vi "Read DIO signals.vi"(8 "error in (no error)":errorcluster) -> (0 "error out":errorcluster, 3 "Relays":T1)   [LabVIEW 2025]
uses:
  Controls/DUT_Relays.ctl
  Controls/CHMB_Relays.ctl
  Controls/Relays.ctl
  <vilib>/Utility/config.llb/Read Key (U32).vi
  <vilib>/Utility/config.llb/NI_LVConfig.lvlib
panel:
  out "CHMB2":T2
  out "CHMB1":T2
  out "DUT4":T3
  out "DUT3":T3
  out "DUT2":T3
  out "DUT1":T3
  out "error IO":errorcluster
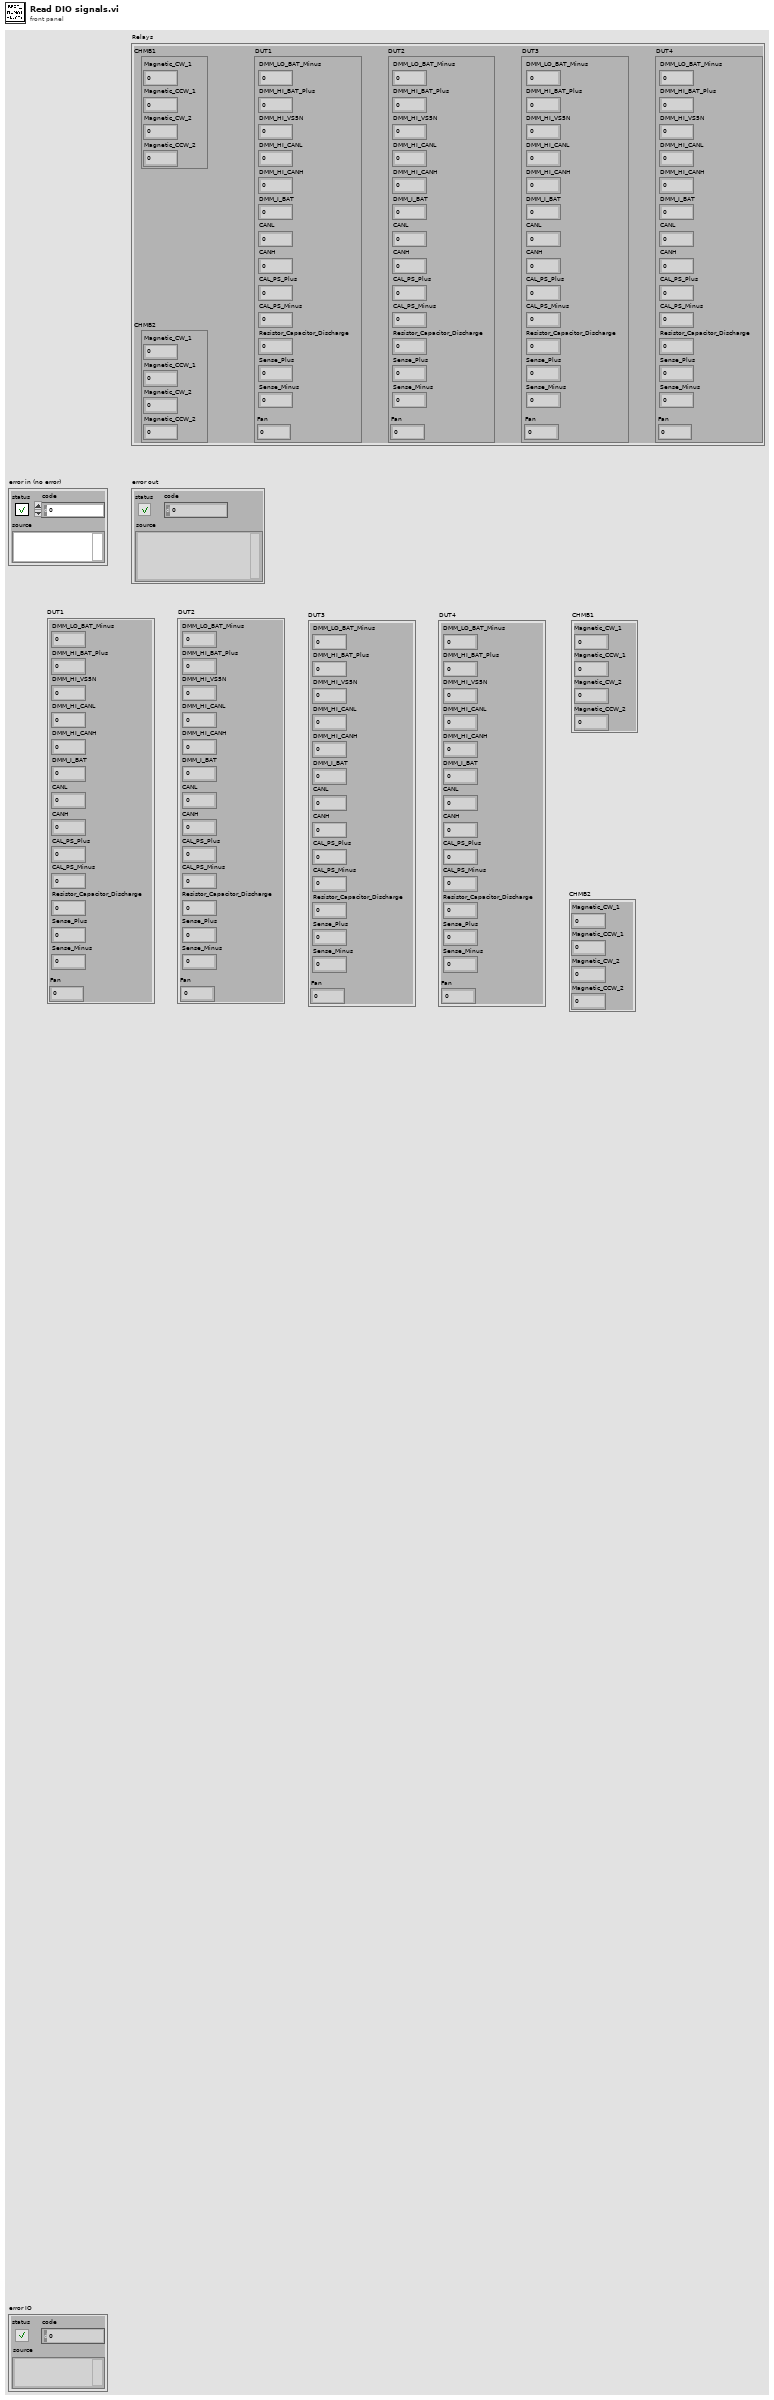
[diagram p1: front panel]
types:
  T1 = typedef "Relays.ctl" = cluster{"CHMB1":T2, "CHMB2":T2, "DUT1":T3, "DUT2":T3, "DUT3":T3, "DUT4":T3}
  T2 = typedef "CHMB_Relays.ctl" = cluster{"Magnetic_CW_1":i32, "Magnetic_CCW_1":i32, "Magnetic_CW_2":i32, "Magnetic_CCW_2":i32}
  T3 = typedef "DUT_Relays.ctl" = cluster{"DMM_LO_BAT_Minus":i32, "DMM_HI_BAT_Plus":i32, "DMM_HI_VS5N":i32, "DMM_HI_CANL":i32, "DMM_HI_CANH":i32, "DMM_I_BAT":i32, "CANL":i32, "CANH":i32, "CAL_PS_Plus":i32, "CAL_PS_Minus":i32, "Resistor_Capacitor_Discharge":i32, "Sense_Plus":i32, "Sense_Minus":i32, "Fan":i32}
  T4 = typedef "NI_LVConfig.lvlib/Config Data RefNum.ctl" = refnum<k1>
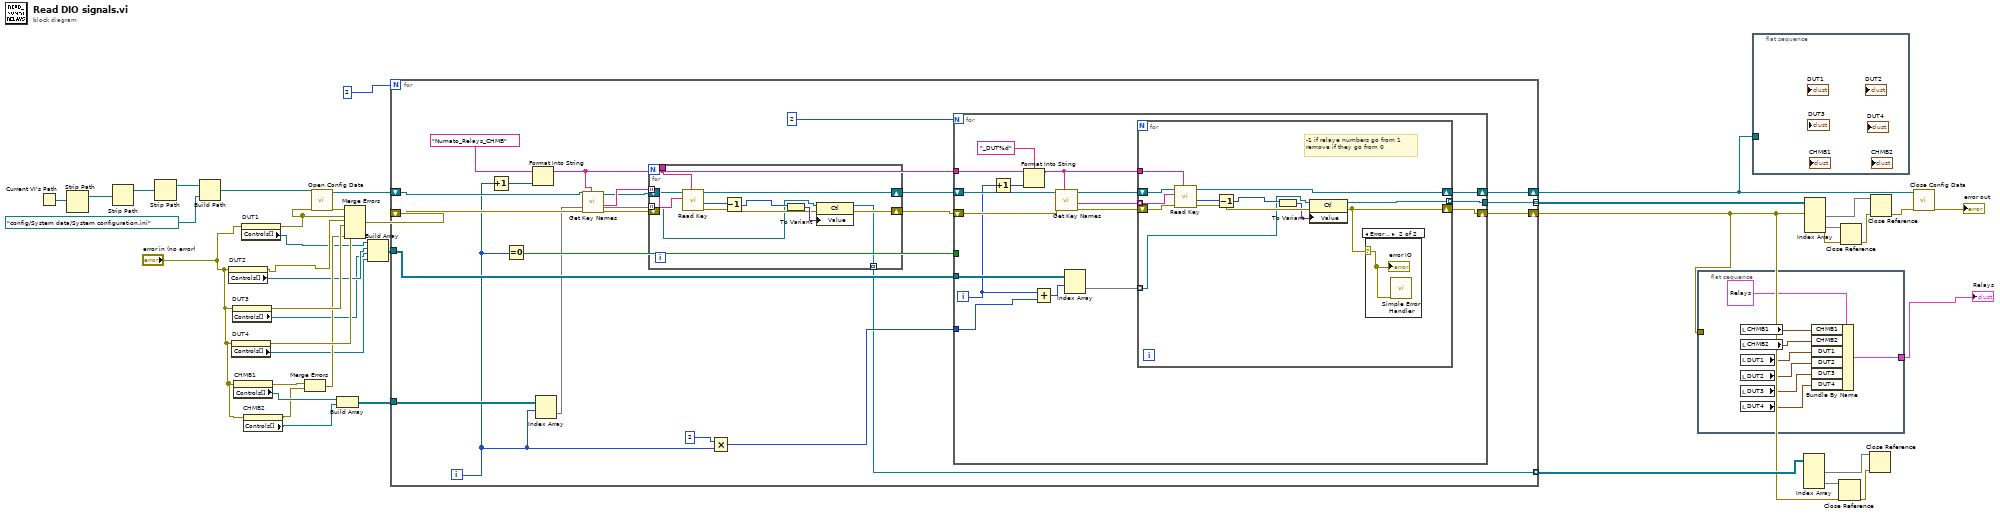
[diagram p0: block diagram]
diagram:
  n1 = Current VI's Path() -> (path=w26:path)
  n2 = Strip Path(path=w26) -> (stripped path=w25:path)  [unwired: 1 out]
  n3 = Strip Path(path=w25) -> (stripped path=w29:path)  [unwired: 1 out]
  n4 = Strip Path(path=w29) -> (stripped path=w28:path)  [unwired: 1 out]
  n5 = Build Path(base path=w28, name or relative path=path "config/System data/System configuration.ini") -> (appended path=w24:path)
  n6 = property on="DUT2" class="Clust (strict)"(error in="error in (no error)") -> (error out=w22:errorcluster, "Controls[]"=w16:refnum<vi>[])  [unwired: 1 in, 1 out]
  n7 = property on="DUT4" class="Clust (strict)"(error in="error in (no error)") -> (error out=w19:errorcluster, "Controls[]"=w14:refnum<vi>[])  [unwired: 1 in, 1 out]
  n8 = property on="DUT3" class="Clust (strict)"(error in="error in (no error)") -> (error out=w20:errorcluster, "Controls[]"=w15:refnum<vi>[])  [unwired: 1 in, 1 out]
  n9 = property on="CHMB1" class="Clust (strict)"(error in="error in (no error)") -> (error out=w21:errorcluster, "Controls[]"=w12:refnum<vi>[])  [unwired: 1 in, 1 out]
  n10 = property on="DUT1" class="Clust (strict)"(error in="error in (no error)") -> (error out=w23:errorcluster, "Controls[]"=w17:refnum<vi>[])  [unwired: 1 in, 1 out]
  n11 = property on="CHMB2" class="Clust (strict)"(error in="error in (no error)") -> (error out=w5:errorcluster, "Controls[]"=w4:refnum<vi>[])  [unwired: 1 in, 1 out]
  n12 = Merge Errors(w21, w5) -> (w18:errorcluster)
  n13 = call <vilib>:"Open Config Data.vi"("error in (no error)"=w23, "configuration file path"=w24) -> ("error out"=w34:errorcluster, "refnum"=w39:T4)  [unwired: 7 in, 1 out]
  n14 = Build Array(w12, w4) -> (w11:refnum<vi>[][])
  n15 = Merge Errors(w34, w23, w22, w20, w19, w18) -> (w35:errorcluster)
  n16 = Build Array(w17, w16, w15, w14) -> (w13:refnum<vi>[][])
  n17 = for {
    N: 2 -> [_]
    shift-right: [w60] -> w3
    shift-left: w39 -> [w55]
    shift-right: [w61] -> w2
    shift-left: w35 -> [w54]
    tunnel: [w57] -> w33 mode=indexing
    tunnel: w13 -> [w52]
    tunnel: w11 -> [w50]
    tunnel: [w41] -> w10 mode=indexing
    i -> [w40]
    n18 = Increment(x=w40) -> (x+1=w51:i32)
    n19 = Equal To 0?(x=w40) -> (x = 0?=w58:bool)
    n20 = Format Into String(initial string="Numato_Relays_CHMB" ("section"), w51) -> (resulting string=w46:string)  [unwired: 2 in, 1 out]
    n21 = Index Array(array=w50, index (row)=w40) -> (element=w49:refnum<vi>[])  [unwired: 1 in]
    n22 = call <vilib>:"Get Key Names.vi"("section"=w46, "error in (no error)"=w54, "refnum"=w55) -> ("error out"=w44:errorcluster, "key names"=w53:string[], "refnum out"=w43:T4)  [unwired: 5 in, 1 out]
    n23 = for {
      tunnel: w53 -> [w68] mode=indexing
      tunnel: w49 -> [w66] mode=indexing
      tunnel: w46 -> [w67]
      shift-right: [w65] -> w45
      shift-left: w44 -> [_]
      shift-right: [w63] -> w42
      shift-left: w43 -> [w64]
      tunnel: [w62] -> w41 mode=indexing
      n24 = call-poly <vilib>:"Read Key.vi"("section"=w67, "key"=w68, "refnum"=w64) -> ("error out"=w69:errorcluster, "value"=w70:u32, "refnum out"=w63:T4)  [unwired: 5 in, 1 out]
      n25 = Decrement(x=w70) -> (x-1=w71:u32)
      n26 = To Variant(anything=w71) -> (Variant=w72:variant)
      n27 = property class="Ctl"(reference=w66, error in=w69, "Value"=w72) -> (reference out=w62:refnum<vi>, error out=w65:errorcluster)
    }
    n28 = Multiply(x=2, y=w40) -> (x*y=w47:i32)
    n29 = for {
      N: 2 -> [_]
      tunnel: w58 -> [_]
      tunnel: [w83] -> w57
      shift-right: [w84] -> w60
      shift-left: w42 -> [w89]
      shift-right: [w85] -> w61
      shift-left: w45 -> [w87]
      tunnel: w46 -> [w81]
      tunnel: w52 -> [w78]
      tunnel: w47 -> [w75]
      i -> [w73]
      n30 = Increment(x=w73) -> (x+1=w76:i32)
      n31 = Format Into String(format string="_DUT%d", initial string=w81, w76) -> (resulting string=w80:string)  [unwired: 1 in, 1 out]
      n32 = Add(x=w73, y=w75) -> (x+y=w74:i32)
      n33 = call <vilib>:"Get Key Names.vi"("section"=w80, "error in (no error)"=w87, "refnum"=w89) -> ("error out"=w86:errorcluster, "key names"=w82:string[], "refnum out"=w88:T4)  [unwired: 5 in, 1 out]
      n34 = Index Array(array=w78, index (row)=w74) -> (element=w77:refnum<vi>[])  [unwired: 1 in]
      n35 = for {
        tunnel: w82 -> [w99] mode=indexing
        shift-right: [w100] -> w84
        shift-left: w88 -> [w101]
        tunnel: w80 -> [w98]
        tunnel: [w95] -> w83 mode=indexing
        shift-right: [w94] -> w85
        shift-left: w86 -> [w97]
        tunnel: w77 -> [w91] mode=indexing
        # "-1 if relaye numbers go from 1\nremove if they go from 0"
        n36 = call-poly <vilib>:"Read Key.vi"("section"=w98, "error in (no error)"=w97, "key"=w99, "refnum"=w101) -> ("error out"=w96:errorcluster, "value"=w93:u32, "refnum out"=w100:T4)  [unwired: 4 in, 1 out]
        n37 = Decrement(x=w93) -> (x-1=w92:u32)
        n38 = To Variant(anything=w92) -> (Variant=w90:variant)
        n39 = property class="Ctl"(reference=w91, error in=w96, "Value"=w90) -> (reference out=w95:refnum<vi>, error out=w94:errorcluster)
        n40 = case shown="Error .." w94 {
          selector: w94 -> [_ w102]
          frame No Error {
          }
          frame Error {
            n41 = call <vilib>:"Simple Error Handler.vi"("error in (no error)"=w102) -> ()  [unwired: 4 in, 5 out]
            "error IO" <- w102
          }
        }
      }
    }
  }
  n42 = flat-sequence {
    tunnel: w2 -> [_]
    tunnel: [w104] -> w1
    frame #0 {
      n43 = local read "CHMB1"() -> (w109:T2)
      n44 = local read "CHMB2"() -> (w103:T2)
      n45 = local read "DUT1"() -> (w108:T3)
      n46 = local read "DUT2"() -> (w107:T3)
      n47 = local read "DUT3"() -> (w106:T3)
      n48 = local read "DUT4"() -> (w105:T3)
      n49 = Bundle By Name(cluster=T1 {"CHMB1"={"Magnetic_CW_1"=0, "Magnetic_CCW_1"=0, "Magnetic_CW_2"=0, "Magnetic_CCW_2"=0}, "CHMB2"={"Magnetic_CW_1"=0, "Magnetic_CCW_1"=0, "Magnetic_CW_2"=0, "Magnetic_CCW_2"=0}, "DUT1"={"DMM_LO_BAT_Minus"=0, "DMM_HI_BAT_Plus"=0, "DMM_HI_VS5N"=0, "DMM_HI_CANL"=0, "DMM_HI_CANH"=0, "DMM_I_BAT"=0, "CANL"=0, "CANH"=0, "CAL_PS_Plus"=0, "CAL_PS_Minus"=0, "Resistor_Capacitor_Discharge"=0, "Sense_Plus"=0, "Sense_Minus"=0, "Fan"=0}, "DUT2"={"DMM_LO_BAT_Minus"=0, "DMM_HI_BAT_Plus"=0, "DMM_HI_VS5N"=0, "DMM_HI_CANL"=0, "DMM_HI_CANH"=0, "DMM_I_BAT"=0, "CANL"=0, "CANH"=0, "CAL_PS_Plus"=0, "CAL_PS_Minus"=0, "Resistor_Capacitor_Discharge"=0, "Sense_Plus"=0, "Sense_Minus"=0, "Fan"=0}, "DUT3"={"DMM_LO_BAT_Minus"=0, "DMM_HI_BAT_Plus"=0, "DMM_HI_VS5N"=0, "DMM_HI_CANL"=0, "DMM_HI_CANH"=0, "DMM_I_BAT"=0, "CANL"=0, "CANH"=0, "CAL_PS_Plus"=0, "CAL_PS_Minus"=0, "Resistor_Capacitor_Discharge"=0, "Sense_Plus"=0, "Sense_Minus"=0, "Fan"=0}, "DUT4"={"DMM_LO_BAT_Minus"=0, "DMM_HI_BAT_Plus"=0, "DMM_HI_VS5N"=0, "DMM_HI_CANL"=0, "DMM_HI_CANH"=0, "DMM_I_BAT"=0, "CANL"=0, "CANH"=0, "CAL_PS_Plus"=0, "CAL_PS_Minus"=0, "Resistor_Capacitor_Discharge"=0, "Sense_Plus"=0, "Sense_Minus"=0, "Fan"=0}} ("Relays"), "CHMB1"=w109, "CHMB2"=w103, "DUT1"=w108, "DUT2"=w107, "DUT3"=w106, "DUT4"=w105) -> (w104:T1)
    }
  }
  n50 = flat-sequence {
    tunnel: w3 -> [_]
    frame #0 {
    }
  }
  n51 = Index Array(array=w10) -> (element #1=w7:refnum<vi>[], element #2=w8:refnum<vi>[])  [unwired: 4 in]
  n52 = Index Array(array=w33) -> (element #1=w32:refnum<vi>[], element #2=w31:refnum<vi>[])  [unwired: 4 in]
  n53 = Close Reference(reference=w8, error in (no error)=w2) -> (error out=w9:errorcluster)
  n54 = Close Reference(reference=w31, error in (no error)=w2) -> (error out=w30:errorcluster)
  n55 = Close Reference(reference=w7, error in (no error)=w9) -> ()  [unwired: 1 out]
  n56 = Close Reference(reference=w32, error in (no error)=w30) -> (error out=w38:errorcluster)
  n57 = call <vilib>:"Close Config Data.vi"("error in (no error)"=w38, "refnum"=w3) -> ("error out"=→"error out":errorcluster)  [unwired: 8 in, 1 out]
  "Relays" <- w1
